vi "Global_CMD.vi"() -> ()   [LabVIEW 2017, in "Gimbal.lvlib"]
uses:
  Gimbal.lvlib
  TypeDefs/Cluster_Gimbal CMD.ctl
  TypeDefs/Cluster_Gimbal Axis CMD.ctl
  TypeDefs/ENUM_Gimbal CMD Mode.ctl
panel:
  in  "CMD_Gimbal":T1
  # "The Names of the Data items in the Global Variable MUST describe who the Single Writer is\nNaming Convention for Command Globals is:   \n\nCMD_SubSystem_Data Name\nExample:\nCMD_Drive_Mode\nCMD_Hopper_Fire Ball"
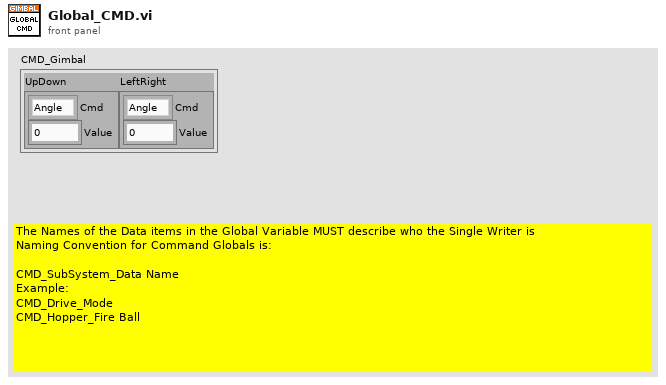
[diagram p1: front panel]
types:
  T1 = typedef "Cluster_Gimbal CMD.ctl" = cluster{"UpDown":T2, "LeftRight":T2}
  T2 = typedef "Cluster_Gimbal Axis CMD.ctl" = cluster{"Cmd":T3, "Value":dbl}
  T3 = typedef "ENUM_Gimbal CMD Mode.ctl" = enum16{"Angle", "Error"}
diagram:
